vi "Read Sensors.vi"(11 "MagnetometerRef":T1={"DevStatus"={"status"=FALSE, "code"=0, "source"=""}, "Controller"=enum."Controller 1", "Device Address"=0, "Handle"=0, "I2C Bus"=enum."Invalid"} {"Device Address" format="%.0x"}) -> ()   [LabVIEW 2014]
uses:
  <vilib>/Rock Robotics/WPI/I2C/WPI_I2CDevRef.ctl
  <vilib>/Rock Robotics/SystemInterfaces/Typedef/FPGA_TypedefDigitalModule.ctl
  <vilib>/Rock Robotics/SystemInterfaces/i2clib/i2c_bus.ctl
  <vilib>/Rock Robotics/WPI/DriverStation/WPI_DriverStationRobotMode2.ctl
  <vilib>/Rock Robotics/Network Tables/SD Read Boolean.vi
  Global Variables/Refnum Names.vi
  Global Variables/Sensor Data (Edited).vi
  Global Variables/Calibrations.vi
  Global Variables/Settings.vi
  Robot Global Data.vi
  Global Variables/Miscalleneous.vi
  <vilib>/Rock Robotics/Network Tables/SD Write Numeric Array.vi
panel:
  out "Left (Outside)":errorcluster
  out "Right (Inside)":errorcluster
  out "Right (Outside)":errorcluster
  out "Left (Inside)":errorcluster
  out "Robot Y":dbl
  out "Robot X":dbl
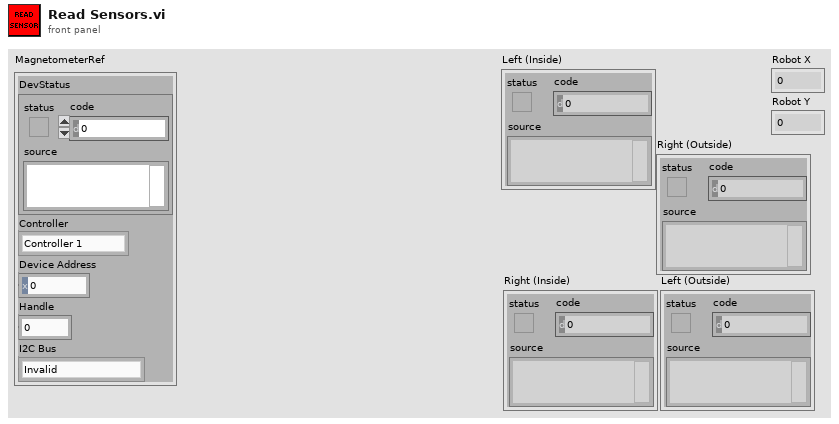
[diagram p1: front panel]
types:
  T1 = typedef "WPI_I2CDevRef.ctl" = cluster{"DevStatus":errorcluster, "Controller":T2, "Device Address":u8, "Handle":i32, "I2C Bus":T3}
  T2 = typedef "FPGA_TypedefDigitalModule.ctl" = enum16{"Controller 1"}
  T3 = typedef "i2c_bus.ctl" = enum16{"I2C On-Board", "I2C MXP", "Invalid"}
  T4 = typedef "WPI_DriverStationRobotMode2.ctl" = enum16{"Autonomous Disabled", "Autonomous Enabled", "Teleop Disabled", "Teleop Enabled", "Disconnected", "Finish", "Test Disabled", "Test Enabled", "Emergency Stopped"}
  T5 = typedef "WPI_EncoderDevRef.ctl" = cluster{"DevStatus":errorcluster, "EncoderIndex":T6, "CounterIndex":T7, "DistancePerCount":dbl, "Decoding Type":T8}
  T6 = typedef "FPGA_EncoderIdx.ctl" = enum8{"Enc 0", "Enc 1", "Enc 2", "Enc 3", "Enc 4", "Enc 5", "Enc 6", "Enc 7", "Invalid"}
  T7 = typedef "FPGA_CounterCtrSystemIndex.ctl" = enum8{"Ctr 0", "Ctr 1", "Ctr 2", "Ctr 3", "Ctr 4", "Ctr 5", "Ctr 6", "Ctr 7", "Invalid"}
  T8 = typedef "WPI_EncoderType.ctl" = enum16{"1x", "2x", "4x"}
  T9 = typedef "WPI_GyroDevRef.ctl" = cluster{"DevStatus":errorcluster, "Analog Module":T10, "Analog Channel":T11, "Offset":dbl, "Gain (VoltsPerDegree/Second)":dbl}
  T10 = typedef "FPGA_TypedefAnalogModule.ctl" = enum16{"Controller 1"}
  T11 = typedef "FPGA_AIChannel.ctl" = enum8{"AI 0", "AI 1", "AI 2", "AI 3", "AI MXP 0", "AI MXP 1", "AI MXP 2", "AI MXP 3", "Invalid"}
  T12 = typedef "WPI_DigitalInputDevRef.ctl" = cluster{"DevStatus":errorcluster, "DIO Channel":T13, "Controller":T2}
  T13 = typedef "FPGA_DIOChannel.ctl" = enum8{"DIO 0", "DIO 1", "DIO 2", "DIO 3", "DIO 4", "DIO 5", "DIO 6", "DIO 7", "DIO 8", "DIO 9", "DIO MXP 0", "DIO MXP 1", "DIO MXP 2", "DIO MXP 3", "DIO MXP 4", "DIO MXP 5", "DIO MXP 6", "DIO MXP 7", "DIO MXP 8", "DIO MXP 9", "DIO MXP 10", "DIO MXP 11", "DIO MXP 12", "DIO MXP 13", "DIO MXP 14", "DIO MXP 15", "Invalid"}
  T14 = typedef "Magnetometer Readings Cluster.ctl" = cluster{"X":i32, "Y":i32, "Z":i32}
  T15 = typedef "Swerve Sensors DevRef.ctl" = cluster{"Front Right Wheel":T16, "Front Left Wheel":T16, "Rear Right Wheel":T16, "Rear Left Wheel":T16}
  T16 = typedef "WPI_AnalogChannelDevRef.ctl" = cluster{"DevStatus":errorcluster, "Controller":T10, "Analog Channel":T11}
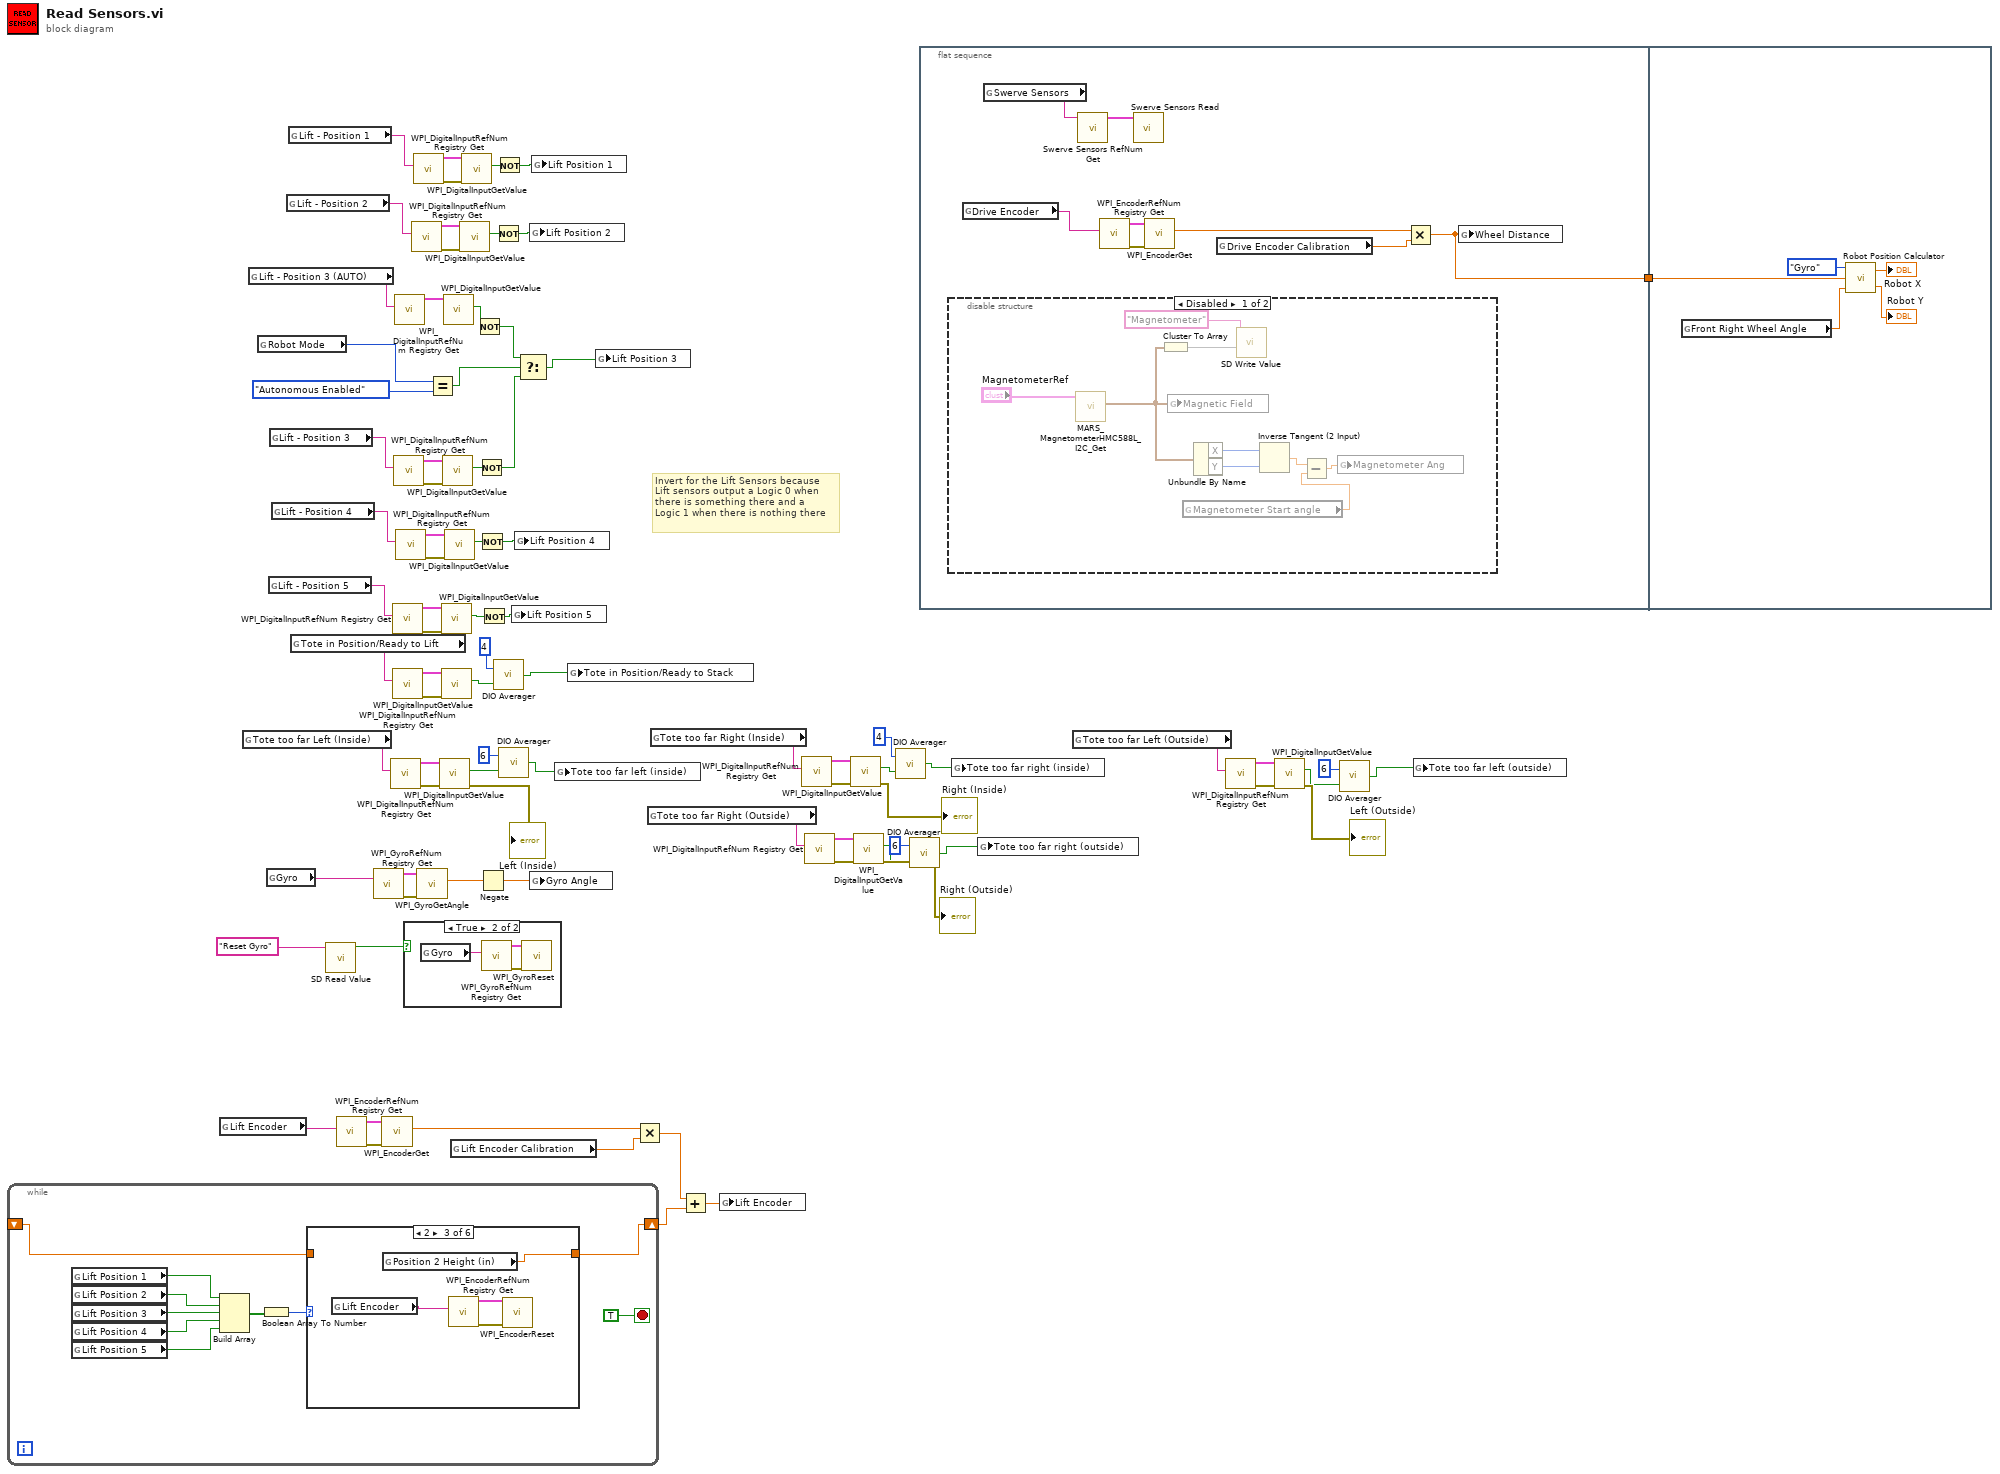
[diagram p0: block diagram]
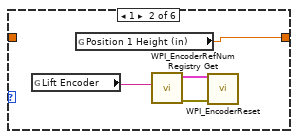
[diagram p4: hidden frame]
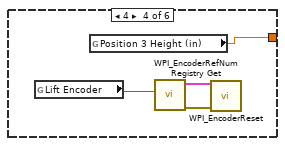
[diagram p5: hidden frame]
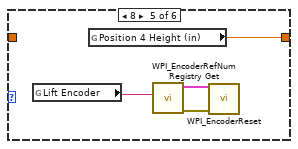
[diagram p6: hidden frame]
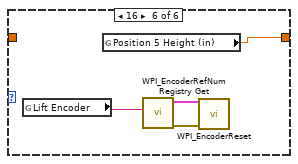
[diagram p7: hidden frame]
diagram:
  # "Invert for the Lift Sensors because\nLift sensors output a Logic 0 when\nthere is something there and a\nLogic 1 when there is nothing there"
  n1 = while {
    shift-right: [w85] -> w45
    shift-left: _ -> [w84]
    stop <- TRUE stop-if-true
    n2 = global read "Sensor Data (Edited).vi" "Lift Position 1"() -> (w86:bool)
    n3 = global read "Sensor Data (Edited).vi" "Lift Position 2"() -> (w87:bool)
    n4 = global read "Sensor Data (Edited).vi" "Lift Position 3"() -> (w88:bool)
    n5 = global read "Sensor Data (Edited).vi" "Lift Position 4"() -> (w89:bool)
    n6 = global read "Sensor Data (Edited).vi" "Lift Position 5"() -> (w90:bool)
    n7 = Build Array(w86, w87, w88, w89, w90) -> (w91:bool[])
    n8 = Boolean Array To Number(Boolean array=w91) -> (number=w92:u32)
    n9 = case shown="2" w92 {
      tunnel: [w94 w95 w99 w103 w107 w111] -> w85
      tunnel: w84 -> [w94 _ _ _ _ _]
      frame 0, Default {
      }
      frame 1 {
        n10 = global read "Refnum Names.vi" "Lift Encoder"() -> (w98:string)
        n11 = global read "Settings.vi" "Position 1 Height (in)"() -> (w95:dbl)
        n12 = call <vilib>:"WPI_EncoderRefNum Registry Get.vi"("refnum name"=w98) -> ("error out"=w97:errorcluster, "EncoderDevRef"=w96:T5)  [unwired: 9 in]
        n13 = call <vilib>:"WPI_EncoderReset.vi"("error in (no error)"=w97, "EncoderDevRef"=w96) -> ()  [unwired: 8 in, 2 out]
      }
      frame 2 {
        n14 = global read "Refnum Names.vi" "Lift Encoder"() -> (w102:string)
        n15 = global read "Settings.vi" "Position 2 Height (in)"() -> (w99:dbl)
        n16 = call <vilib>:"WPI_EncoderRefNum Registry Get.vi"("refnum name"=w102) -> ("error out"=w101:errorcluster, "EncoderDevRef"=w100:T5)  [unwired: 9 in]
        n17 = call <vilib>:"WPI_EncoderReset.vi"("error in (no error)"=w101, "EncoderDevRef"=w100) -> ()  [unwired: 8 in, 2 out]
      }
      frame 4 {
        n18 = global read "Refnum Names.vi" "Lift Encoder"() -> (w106:string)
        n19 = global read "Settings.vi" "Position 3 Height (in)"() -> (w103:dbl)
        n20 = call <vilib>:"WPI_EncoderRefNum Registry Get.vi"("refnum name"=w106) -> ("error out"=w105:errorcluster, "EncoderDevRef"=w104:T5)  [unwired: 9 in]
        n21 = call <vilib>:"WPI_EncoderReset.vi"("error in (no error)"=w105, "EncoderDevRef"=w104) -> ()  [unwired: 8 in, 2 out]
      }
      frame 8 {
        n22 = global read "Refnum Names.vi" "Lift Encoder"() -> (w110:string)
        n23 = global read "Settings.vi" "Position 4 Height (in)"() -> (w107:dbl)
        n24 = call <vilib>:"WPI_EncoderRefNum Registry Get.vi"("refnum name"=w110) -> ("error out"=w109:errorcluster, "EncoderDevRef"=w108:T5)  [unwired: 9 in]
        n25 = call <vilib>:"WPI_EncoderReset.vi"("error in (no error)"=w109, "EncoderDevRef"=w108) -> ()  [unwired: 8 in, 2 out]
      }
      frame 16 {
        n26 = global read "Refnum Names.vi" "Lift Encoder"() -> (w114:string)
        n27 = global read "Settings.vi" "Position 5 Height (in)"() -> (w111:dbl)
        n28 = call <vilib>:"WPI_EncoderRefNum Registry Get.vi"("refnum name"=w114) -> ("error out"=w113:errorcluster, "EncoderDevRef"=w112:T5)  [unwired: 9 in]
        n29 = call <vilib>:"WPI_EncoderReset.vi"("error in (no error)"=w113, "EncoderDevRef"=w112) -> ()  [unwired: 8 in, 2 out]
      }
    }
  }
  n30 = global read "Refnum Names.vi" "Lift Encoder"() -> (w61:string)
  n31 = global read "Refnum Names.vi" "Tote too far Left (Inside)"() -> (w29:string)
  n32 = global read "Refnum Names.vi" "Lift - Position 3 (AUTO)"() -> (w35:string)
  n33 = global read "Robot Global Data.vi" "Robot Mode"() -> (w38:T4)
  n34 = global read "Refnum Names.vi" "Gyro"() -> (w53:string)
  n35 = global read "Refnum Names.vi" "Lift - Position 5"() -> (w65:string)
  n36 = global read "Refnum Names.vi" "Lift - Position 3"() -> (w73:string)
  n37 = global read "Refnum Names.vi" "Lift - Position 4"() -> (w70:string)
  n38 = global read "Refnum Names.vi" "Lift - Position 2"() -> (w78:string)
  n39 = global read "Refnum Names.vi" "Lift - Position 1"() -> (w81:string)
  n40 = global read "Refnum Names.vi" "Tote in Position/Ready to Lift"() -> (w58:string)
  n41 = call-poly <vilib>:"SD Read Value.vi"("Name"="Reset Gyro") -> ("Boolean"=w51:bool)  [unwired: 8 in, 2 out]
  n42 = call <vilib>:"WPI_EncoderRefNum Registry Get.vi"("refnum name"=w61) -> ("error out"=w63:errorcluster, "EncoderDevRef"=w62:T5)  [unwired: 9 in]
  n43 = call <vilib>:"WPI_GyroRefNum Registry Get.vi"("refnum name"=w53) -> ("error out"=w55:errorcluster, "GyroDevRef"=w54:T9)  [unwired: 9 in]
  n44 = call <vilib>:"WPI_EncoderGet.vi"("error in (no error)"=w63, "EncoderDevRef"=w62) -> ("Distance"=w60:dbl)  [unwired: 4 in, 5 out]
  n45 = call <vilib>:"WPI_DigitalInputRefNum Registry Get.vi"("refnum name"=w29) -> ("error out"=w31:errorcluster, "DigitalInputDevRef"=w30:T12)  [unwired: 9 in]
  n46 = call <vilib>:"WPI_DigitalInputRefNum Registry Get.vi"("refnum name"=w65) -> ("error out"=w67:errorcluster, "DigitalInputDevRef"=w66:T12)  [unwired: 9 in]
  n47 = call <vilib>:"WPI_DigitalInputRefNum Registry Get.vi"("refnum name"=w58) -> ("error out"=w56:errorcluster, "DigitalInputDevRef"=w57:T12)  [unwired: 9 in]
  n48 = call <vilib>:"WPI_DigitalInputRefNum Registry Get.vi"("refnum name"=w73) -> ("error out"=w75:errorcluster, "DigitalInputDevRef"=w74:T12)  [unwired: 9 in]
  n49 = call <vilib>:"WPI_DigitalInputRefNum Registry Get.vi"("refnum name"=w35) -> ("DigitalInputDevRef"=w34:T12)  [unwired: 9 in, 1 out]
  n50 = call <vilib>:"WPI_DigitalInputRefNum Registry Get.vi"("refnum name"=w70) -> ("error out"=w68:errorcluster, "DigitalInputDevRef"=w69:T12)  [unwired: 9 in]
  n51 = case shown="True" w51 {
    frame False {
    }
    frame True {
      n52 = global read "Refnum Names.vi" "Gyro"() -> (w115:string)
      n53 = call <vilib>:"WPI_GyroRefNum Registry Get.vi"("refnum name"=w115) -> ("error out"=w116:errorcluster, "GyroDevRef"=w117:T9)  [unwired: 9 in]
      n54 = call <vilib>:"WPI_GyroReset.vi"("error in (no error)"=w116, "GyroDevRef"=w117) -> ()  [unwired: 8 in, 2 out]
    }
  }
  n55 = call <vilib>:"WPI_DigitalInputRefNum Registry Get.vi"("refnum name"=w78) -> ("error out"=w76:errorcluster, "DigitalInputDevRef"=w77:T12)  [unwired: 9 in]
  n56 = call <vilib>:"WPI_DigitalInputRefNum Registry Get.vi"("refnum name"=w81) -> ("error out"=w83:errorcluster, "DigitalInputDevRef"=w82:T12)  [unwired: 9 in]
  n57 = call <vilib>:"WPI_GyroGetAngle.vi"("error in (no error)"=w55, "GyroDevRef"=w54) -> ("Angle"=w46:dbl)  [unwired: 6 in, 3 out]
  n58 = Equal?(x=w38, y=WPI_DriverStationRobotMode2."Autonomous Enabled") -> (x = y?=w36:bool)
  n59 = call <vilib>:"WPI_DigitalInputGetValue.vi"("error in (no error)"=w31, "DigitalInputDevRef"=w30) -> ("error out"=→"Left (Inside)":errorcluster, "Value"=w2:bool)  [unwired: 7 in, 1 out]
  n60 = call <vilib>:"WPI_DigitalInputGetValue.vi"("error in (no error)"=w67, "DigitalInputDevRef"=w66) -> ("Value"=w64:bool)  [unwired: 7 in, 2 out]
  n61 = call <vilib>:"WPI_DigitalInputGetValue.vi"("error in (no error)"=w56, "DigitalInputDevRef"=w57) -> ("Value"=w11:bool)  [unwired: 7 in, 2 out]
  n62 = call <vilib>:"WPI_DigitalInputGetValue.vi"("error in (no error)"=w75, "DigitalInputDevRef"=w74) -> ("Value"=w72:bool)  [unwired: 7 in, 2 out]
  n63 = call <vilib>:"WPI_DigitalInputGetValue.vi"("DigitalInputDevRef"=w34) -> ("Value"=w33:bool)  [unwired: 8 in, 2 out]
  n64 = call <vilib>:"WPI_DigitalInputGetValue.vi"("error in (no error)"=w68, "DigitalInputDevRef"=w69) -> ("Value"=w71:bool)  [unwired: 7 in, 2 out]
  n65 = global read "Calibrations.vi" "Lift Encoder Calibration"() -> (w59:dbl)
  n66 = call <vilib>:"WPI_DigitalInputGetValue.vi"("error in (no error)"=w76, "DigitalInputDevRef"=w77) -> ("Value"=w79:bool)  [unwired: 7 in, 2 out]
  n67 = call <vilib>:"WPI_DigitalInputGetValue.vi"("error in (no error)"=w83, "DigitalInputDevRef"=w82) -> ("Value"=w80:bool)  [unwired: 7 in, 2 out]
  n68 = Not(x=w33) -> (.not. x?=w32:bool)
  n69 = Not(x=w72) -> (.not. x?=w39:bool)
  n70 = Not(x=w71) -> (.not. x?=w48:bool)
  n71 = Negate(x=w46) -> (-x=w42:dbl)
  n72 = Not(x=w64) -> (.not. x?=w47:bool)
  n73 = Not(x=w79) -> (.not. x?=w49:bool)
  n74 = call "DIO Averager.vi"("In"=w11, "Number of Cycles to average"=4) -> ("Out"=w10:bool)
  n75 = Not(x=w80) -> (.not. x?=w50:bool)
  n76 = call "DIO Averager.vi"("In"=w2, "Number of Cycles to average"=6) -> ("Out"=w3:bool)
  n77 = global write "Sensor Data (Edited).vi" "Lift Position 5"(w47) -> ()
  n78 = global write "Sensor Data (Edited).vi" "Lift Position 4"(w48) -> ()
  n79 = Select(t=w32, s=w36, f=w39) -> (s? t:f=w40:bool)
  n80 = global write "Sensor Data (Edited).vi" "Lift Position 2"(w49) -> ()
  n81 = global write "Sensor Data (Edited).vi" "Gyro Angle"(w42) -> ()
  n82 = global write "Sensor Data (Edited).vi" "Lift Position 1"(w50) -> ()
  n83 = global write "Sensor Data (Edited).vi" "Tote too far left (inside)"(w3) -> ()
  n84 = global write "Sensor Data (Edited).vi" "Tote in Position/Ready to Stack"(w10) -> ()
  n85 = global write "Sensor Data (Edited).vi" "Lift Position 3"(w40) -> ()
  n86 = Multiply(x=w60, y=w59) -> (x*y=w44:dbl)
  n87 = global read "Refnum Names.vi" "Tote too far Right (Outside)"() -> (w23:string)
  n88 = global read "Refnum Names.vi" "Tote too far Right (Inside)"() -> (w28:string)
  n89 = Add(x=w44, y=w45) -> (x+y=w43:dbl)
  n90 = global write "Sensor Data (Edited).vi" "Lift Encoder"(w43) -> ()
  n91 = call <vilib>:"WPI_DigitalInputRefNum Registry Get.vi"("refnum name"=w28) -> ("error out"=w26:errorcluster, "DigitalInputDevRef"=w27:T12)  [unwired: 9 in]
  n92 = call <vilib>:"WPI_DigitalInputRefNum Registry Get.vi"("refnum name"=w23) -> ("error out"=w25:errorcluster, "DigitalInputDevRef"=w24:T12)  [unwired: 9 in]
  n93 = call <vilib>:"WPI_DigitalInputGetValue.vi"("error in (no error)"=w26, "DigitalInputDevRef"=w27) -> ("error out"=→"Right (Inside)":errorcluster, "Value"=w5:bool)  [unwired: 7 in, 1 out]
  n94 = call <vilib>:"WPI_DigitalInputGetValue.vi"("error in (no error)"=w25, "DigitalInputDevRef"=w24) -> ("error out"=→"Right (Outside)":errorcluster, "Value"=w15:bool)  [unwired: 7 in, 1 out]
  n95 = call "DIO Averager.vi"("In"=w5, "Number of Cycles to average"=4) -> ("Out"=w6:bool)
  n96 = call "DIO Averager.vi"("In"=w15, "Number of Cycles to average"=6) -> ("Out"=w14:bool)
  n97 = flat-sequence {
    tunnel: [w118] -> w41
    tunnel: w41 -> [w136]
    frame #0 {
      n98 = disable-structure shown="Disabled" {
        frame Disabled {
          n99 = call "MARS_MagnetometerHMC588L_I2C_Get.vi"("I2CDevRef"="MagnetometerRef") -> ("Magnetometer Reading"=w131:T14)  [unwired: 8 in, 2 out]
          n100 = Cluster To Array(cluster=w131) -> (array=w128:i32[])
          n101 = global write "Sensor Data (Edited).vi" "Magnetic Field"(w131) -> ()
          n102 = global read "Miscalleneous.vi" "Magnetometer Start angle"() -> (w133:dbl)
          n103 = Unbundle By Name(w131) -> ("X"=w130:i32, "Y"=w126:i32)
          n104 = call-poly <vilib>:"SD Write Value.vi"("Numeric Array"=w128, "Name"="Magnetometer") -> ()  [unwired: 8 in, 2 out]
          n105 = Inverse Tangent (2 Input)(1:w126, 2:w130) -> (0:w132:dbl)
          n106 = Subtract(x=w132, y=w133) -> (x-y=w134:dbl)
          n107 = global write "Sensor Data (Edited).vi" "Magnetometer Ang"(w134) -> ()
        }
        frame Enabled {
        }
      }
      n108 = global read "Refnum Names.vi" "Drive Encoder"() -> (w121:string)
      n109 = global read "Refnum Names.vi" "Swerve Sensors"() -> (w125:string)
      n110 = call "Swerve Sensors RefNum Get.vi"("Swerve Sensors RefNum"=w125) -> ("Swerve Sensors DevRef"=w124:T15)  [unwired: 10 in]
      n111 = call <vilib>:"WPI_EncoderRefNum Registry Get.vi"("refnum name"=w121) -> ("error out"=w119:errorcluster, "EncoderDevRef"=w120:T5)  [unwired: 9 in]
      n112 = call "Swerve Sensors Read.vi"("Swerve Motor DevRef"=w124) -> ()  [unwired: 11 in]
      n113 = call <vilib>:"WPI_EncoderGet.vi"("error in (no error)"=w119, "EncoderDevRef"=w120) -> ("Distance"=w122:dbl)  [unwired: 4 in, 5 out]
      n114 = global read "Calibrations.vi" "Drive Encoder Calibration"() -> (w123:dbl)
      n115 = Multiply(x=w122, y=w123) -> (x*y=w118:dbl)
      n116 = global write "Sensor Data (Edited).vi" "Wheel Distance"(w118) -> ()
    }
    frame #1 {
      n117 = global read "Sensor Data (Edited).vi" "Front Right Wheel Angle"() -> (w137:dbl)
      n118 = call "Robot Position Calculator.vi"("Current wheel Angle"=w137, "Wheel Encoder"=w136, "Robot Angle Source"=enum16{"Gyro", "Magnetometer", "Kalman Filter"}."Gyro") -> ("Robot Y"=→"Robot Y":dbl, "Robot X"=→"Robot X":dbl)
    }
  }
  n119 = global write "Sensor Data (Edited).vi" "Tote too far right (inside)"(w6) -> ()
  n120 = global write "Sensor Data (Edited).vi" "Tote too far right (outside)"(w14) -> ()
  n121 = global read "Refnum Names.vi" "Tote too far Left (Outside)"() -> (w22:string)
  n122 = call <vilib>:"WPI_DigitalInputRefNum Registry Get.vi"("refnum name"=w22) -> ("error out"=w20:errorcluster, "DigitalInputDevRef"=w21:T12)  [unwired: 9 in]
  n123 = call <vilib>:"WPI_DigitalInputGetValue.vi"("error in (no error)"=w20, "DigitalInputDevRef"=w21) -> ("error out"=→"Left (Outside)":errorcluster, "Value"=w13:bool)  [unwired: 7 in, 1 out]
  n124 = call "DIO Averager.vi"("In"=w13, "Number of Cycles to average"=6) -> ("Out"=w12:bool)
  n125 = global write "Sensor Data (Edited).vi" "Tote too far left (outside)"(w12) -> ()
